vi "MFCclient.vi"(9 "Setpoint":dbl(slide) max=100.0 step=10.0 scale=0.0..100.0, 10 "Valve":bool, 11 "MFCbasename":string) -> ()   [LabVIEW 2016]
panel:
  out "SPComments":string
  out "ValveComments":string
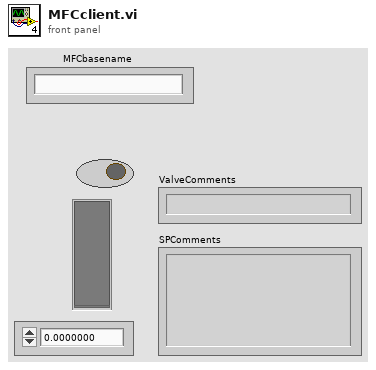
[diagram p1: front panel]
types:
  T1 = typedef "Ch_description_ADAM.ctl" = cluster{"Ch Name":string, "Type":T2, "Function":T3, "Ch State":T4, "Calibration type":T5, "A":dbl, "B":dbl, "C":dbl, "D":dbl, "Comments":string, "Address":T6, "String":string, "Duty":u16}
  T2 = typedef "Module_type_ADAM.ctl" = string
  T3 = typedef "Function_ADAM.ctl" = enum16{"Analogue Input", "Digital Input", "Event counter", "Event rate", "Analogue Output", "Digital Output", "Relay Output"}
  T4 = typedef "Channel_State.ctl" = enum16{"On", "Off", "Always On", "Always Off"}
  T5 = typedef "Calib_type_ADAM.ctl" = string
  T6 = typedef "Address.ctl" = cluster{"Main":i32, "Ch.":i32, "Sub":i32, "Port Name":string}
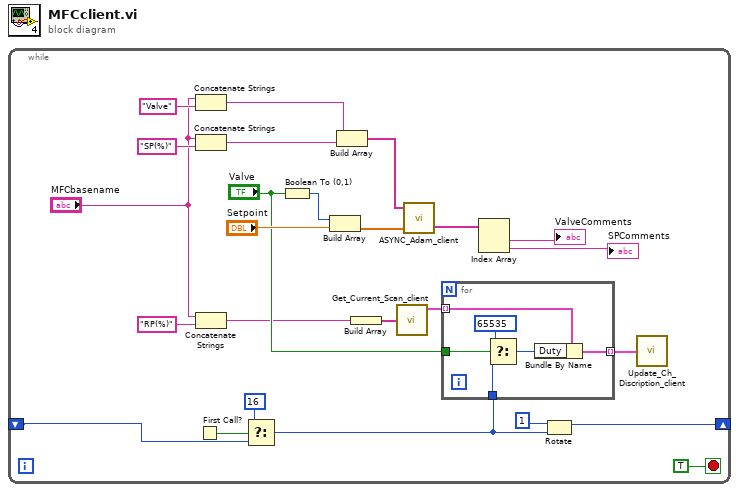
[diagram p0: block diagram]
diagram:
  n1 = while {
    shift-right: [w7] -> _
    shift-left: _ -> [w4]
    stop <- TRUE stop-if-true
    n2 = First Call?() -> (First Call?: T/F=w5:bool)
    n3 = Concatenate Strings("MFCbasename", "Valve" ("string")) -> (w9:string)
    n4 = Concatenate Strings("MFCbasename", "SP(%)" ("string")) -> (w10:string)
    n5 = Concatenate Strings("MFCbasename", "RP(%)" ("string")) -> (w8:string)
    n6 = Select(t=u16 16, s=w5, f=w4) -> (s? t:f=w3:u16)
    n7 = Boolean To (0,1)(Boolean="Valve") -> (0, 1=w23:i16)
    n8 = Build Array(w23, "Setpoint") -> (w25:dbl[])
    n9 = Build Array(w9, w10) -> (w24:string[])
    n10 = Build Array(w8) -> (w18:string[])
    n11 = call "Get_Current_Scan_client.vi"("ADAM Ch Names"=w18) -> ("Ch Description Array"=w17:T1[])  [unwired: 3 out]
    n12 = call "ASYNC_Adam_client.vi"("Values"=w25, "Channel Names"=w24) -> ("Scan Comments"=w21:string[])  [unwired: 1 in, 1 out]
    n13 = for {
      tunnel: w17 -> [w31] mode=indexing
      tunnel: [w30] -> w16 mode=indexing
      tunnel: "Valve" -> [w28]
      tunnel: w3 -> [w26]
      n14 = Select(t=u16 65535 ("Duty"), s=w28, f=w26) -> (s? t:f=w27:u16)
      n15 = Bundle By Name(cluster=w31, "Duty"=w27) -> (w30:T1)
    }
    n16 = Index Array(array=w21) -> (element #1=→"ValveComments":string, element #2=→"SPComments":string)  [unwired: 2 in]
    n17 = Rotate(1:w3, 2:u16 1 ("f")) -> (0:w7:u16)
    n18 = call "Update_Ch_Discription_client.vi"("Channels to update In"=w16) -> ()  [unwired: 1 out]
  }
